vi "Reset.vi"(8 "error in (no error)":errorcluster, 11 "VISA resource name":refnum<visa-resource-name>) -> (0 "error out":errorcluster, 3 "VISA resource name out":refnum<visa-resource-name>)   [LabVIEW 2012, in "Zaber A Series.lvlib"]
doc: "Resets the device. Resetting is equivalent to cycling the power. \n\nThis VI requires that the Initialize VI has been called with the same serial port."
uses:
  <instrlib>/Zaber A Series/Zaber A Series.lvlib
  <instrlib>/Zaber A Series/Private/All Commands.ctl
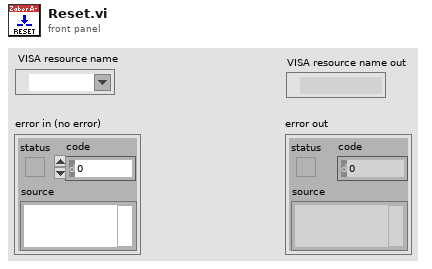
[diagram p1: front panel]
types:
  T1 = typedef "Zaber A Series.lvlib/All Commands.ctl" = string
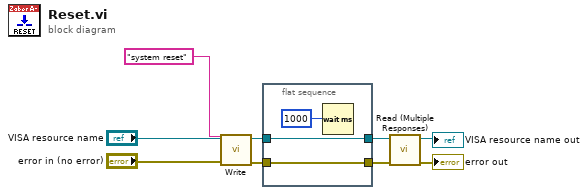
[diagram p0: block diagram]
diagram:
  n1 = call <instrlib>:"Write.vi"("error in (no error)"="error in (no error)", "Command"=T1 "system reset" ("Reset Command"), "VISA resource name"="VISA resource name") -> ("error out"=w4:errorcluster, "VISA resource name out"=w6:refnum<visa-resource-name>)  [unwired: 7 in]
  n2 = flat-sequence {
    tunnel: w6 -> [w12]
    tunnel: [w12] -> w5
    tunnel: w4 -> [w11]
    tunnel: [w11] -> w3
    frame #0 {
      n3 = Wait (ms)(milliseconds to wait=u32 1000) -> ()  [unwired: 1 out]
    }
  }
  n4 = call <instrlib>:"Read (Multiple Responses).vi"("error in (no error)"=w3, "VISA resource name"=w5) -> ("error out"=→"error out":errorcluster, "VISA resource name out"=→"VISA resource name out":refnum<visa-resource-name>)  [unwired: 5 in, 3 out]
